vi "Get Variant Boxed Type Data Size.vi"(8 "error in (no error)":errorcluster, 11 "Data String":u8[](array[numeric])) -> (0 "error out":errorcluster, 2 "Data Size":i32, 3 "Remaining Data String":u8[](array[numeric]))   [LabVIEW 2017, in "Composition.lvlib"]
doc: "Determines the data size of the boxed type inside a variant.\n\n<B>Data Layout</B>\n[version][TD count][TDs][backref count][boxed data][number of attributes][attribute data][...]\n\nThe version part consists of four bytes, where the first part indicates the major LabVIEW version in Hexadecimal (e.g., [0x17, 0x00] = 2017) and the second part for the minor version of LabVIEW (e.g., [0x7f, 0x00] = SP1).\n\nTD count is four bytes indicating how many type definitions are packed in this variant part. What follows are the TDs, where the order of the TD in the set is important because TDs are re-used by index on the main type. For example, a cluster may have two strings. The string type only appears once and is referenced by the cluster twice. Note that types are always referenced, even if they are only used once.\n\nAfter the TDs, there are two bytes which (presumably) return the number of top-level types (so far, only 0x0001 was observed). After this comes the number of backref TDs (e.g., 0x0001 for the previous example of two strings in one cluster).\n\nThe backref TDs must be resolved in the primary TD to receive the \"original\" TD back. Effectively, uncompressing the variant. Here it is important to replace TDs at the right places in the primary TD (always from last to first to avoid replacing actual data).\n\nThe output of this is the unpacked type(s), which are passed as if they have been passed unpacked.\n\nNote that the same logic is used for attributes itself - recursively because an attribute can be a variant with attributes and so forth."
uses:
  Composition.lvlib
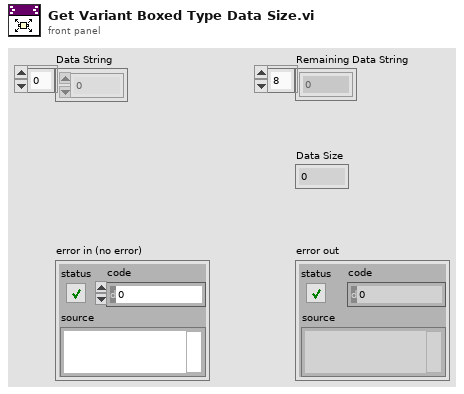
[diagram p1: front panel]
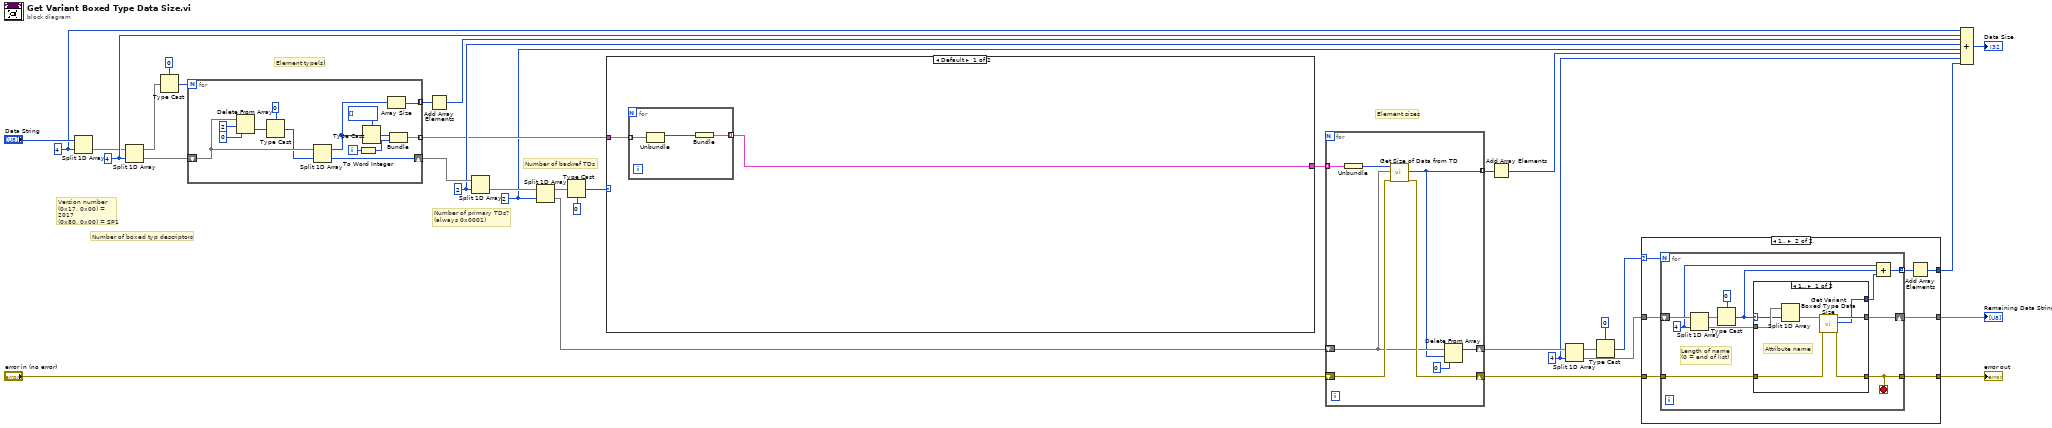
[diagram p0: block diagram]
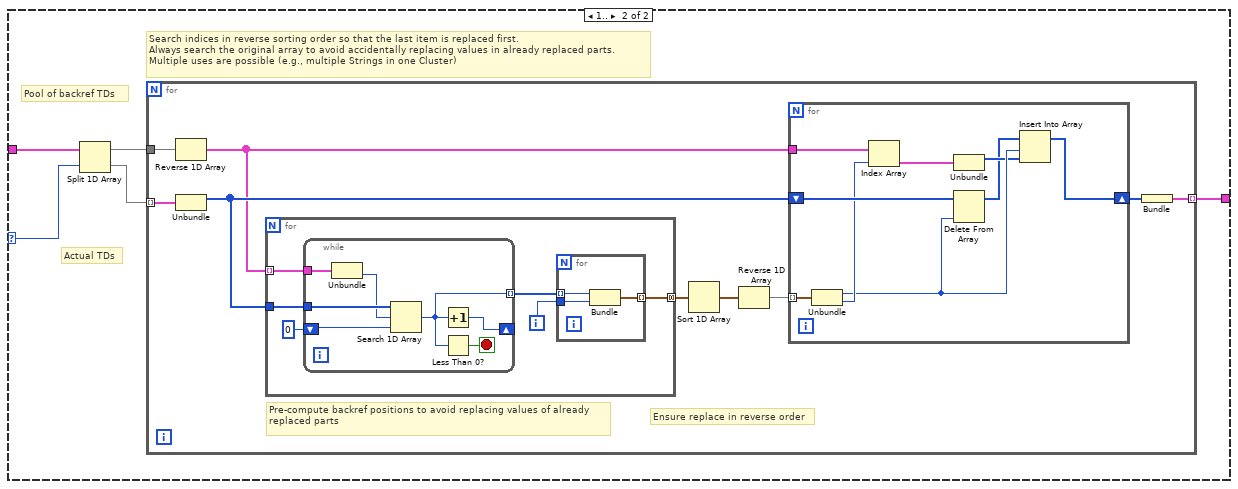
[diagram p4: hidden frame]
diagram:
  w8 = 4 ("index")
  w12 = 2 ("index")
  w26 = 2 ("length")
  w27 = 4 ("length")
  w28 = 4 ("length")
  # "Element sizes"
  # "Number of primary TDs?\n(always 0x0001)"
  # "Number of backref TDs"
  # "Version number\n(0x17, 0x00) = 2017\n(0x80, 0x00) = SP1"
  # "Element type(s)"
  # "Number of boxed typ descriptors"
  n1 = Split 1D Array(array="Data String", index=w28) -> (second subarray=w18:u8[])  [unwired: 1 out]
  n2 = Split 1D Array(array=w18, index=w27) -> (first subarray=w20:u8[], second subarray=w19:u8[])
  n3 = Type Cast(type=0 ("index"), x=w20) -> (*(type *) &x=w31:i32)
  n4 = for {
    N: w31 -> [_]
    shift-right: [w36] -> w30
    shift-left: w19 -> [w45]
    tunnel: [w42] -> w22 mode=indexing
    tunnel: [w39] -> w25 mode=indexing
    i -> [w38]
    n5 = Delete From Array(array=w45, length=2, index=0) -> (deleted portion=w47:u8[])  [unwired: 1 out]
    n6 = Type Cast(type=i16 0 ("index"), x=w47) -> (*(type *) &x=w44:i16)
    n7 = Split 1D Array(array=w45, index=w44) -> (first subarray=w35:u8[], second subarray=w36:u8[])
    n8 = To Word Integer(number=w38) -> (16bit integer=w37:i16)
    n9 = Type Cast(type=i16[] [] ("index"), x=w35) -> (*(type *) &x=w41:i16[])
    n10 = Array Size(array=w35) -> (size(s)=w39:i32)
    n11 = Bundle("index"=w41, w37) -> (w42:cluster{"index":i16[], i16})  [unwired: 1 in]
  }
  n12 = Add Array Elements(numeric array=w25) -> (sum=w24:i32)
  n13 = Split 1D Array(array=w30, index=w26) -> (second subarray=w15:u8[])  [unwired: 1 out]
  n14 = Split 1D Array(array=w15, index=w12) -> (first subarray=w13:u8[], second subarray=w14:u8[])
  n15 = Type Cast(type=i16 0 ("index"), x=w13) -> (*(type *) &x=w21:i16)
  n16 = case shown="Default" w21 {
    selector: w21 -> [_ w54]
    tunnel: w22 -> [w50 w58]
    tunnel: [w49 w55] -> w11
    frame Default {
      n17 = for {
        tunnel: w50 -> [w53] mode=indexing
        tunnel: [w51] -> w49 mode=indexing
        n18 = Unbundle(w53) -> ("index"=w52:i16[])  [unwired: 1 out]
        n19 = Bundle("index"=w52) -> (w51:cluster{"index":i16[]})  [unwired: 1 in]
      }
    }
    frame 1.. {
      # "Search indices in reverse sorting order so that the last item is replaced first.\nAlways search the original array to avoid accidentally replacing values in already replaced parts.\nMultiple uses are possible (e.g., multiple Strings in one Cluster)"
      # "Actual TDs"
      # "Pool of backref TDs"
      n20 = Split 1D Array(array=w58, index=w54) -> (first subarray=w56:cluster{"index":i16[], i16}[], second subarray=w57:cluster{"index":i16[], i16}[])
      n21 = for {
        tunnel: w57 -> [w66] mode=indexing
        tunnel: w56 -> [w67]
        tunnel: [w65] -> w55 mode=indexing
        # "Ensure replace in reverse order"
        # "Pre-compute backref positions to avoid replacing values of already replaced parts"
        n22 = Reverse 1D Array(array=w67) -> (reversed array=w62:cluster{"index":i16[], i16}[])
        n23 = Unbundle(w66) -> ("index"=w63:i16[])  [unwired: 1 out]
        n24 = for {
          tunnel: w62 -> [w72] mode=indexing
          tunnel: w63 -> [w73]
          tunnel: [w69] -> w61 mode=concatenating
          i -> [w70]
          n25 = while {
            tunnel: w73 -> [w83]
            tunnel: w72 -> [w82]
            tunnel: [w78] -> w71 mode=indexing
            shift-right: [w77] -> _
            shift-left: 0 -> [w79]
            stop <- w80 stop-if-true
            n26 = Unbundle(w82) -> (w81:i16)  [unwired: 1 out]
            n27 = Search 1D Array(1D array=w83, element=w81, start index (0)=w79) -> (index of element=w78:i32)
            n28 = Increment(x=w78) -> (x+1=w77:i32)
            n29 = Less Than 0?(x=w78) -> (x < 0?=w80:bool)
          }
          n30 = for {
            tunnel: w71 -> [w75] mode=indexing
            tunnel: w70 -> [w74]
            tunnel: [w76] -> w69 mode=indexing
            n31 = Bundle("index of element"=w75, w74) -> (w76:cluster{"index of element":i32, i32})  [unwired: 1 in]
          }
        }
        n32 = Sort 1D Array(array=w61) -> (sorted array=w60:cluster{"index of element":i32, i32}[])
        n33 = Reverse 1D Array(array=w60) -> (reversed array=w59:cluster{"index of element":i32, i32}[])
        n34 = for {
          tunnel: w62 -> [w89]
          shift-right: [w91] -> w64
          shift-left: w63 -> [w92]
          tunnel: w59 -> [w90] mode=indexing
          n35 = Unbundle(w90) -> ("index of element"=w86:i32, w87:i32)
          n36 = Index Array(array=w89, index=w87) -> (element=w88:cluster{"index":i16[], i16})
          n37 = Unbundle(w88) -> ("index"=w85:i16[])  [unwired: 1 out]
          n38 = Delete From Array(array=w92, index=w86) -> (array with subset deleted=w84:i16[])  [unwired: 1 in, 1 out]
          n39 = Insert Into Array(array=w84, index=w86, new element=w85) -> (w91:i16[])
        }
        n40 = Bundle("index"=w64) -> (w65:cluster{"index":i16[]})  [unwired: 1 in]
      }
    }
  }
  n41 = for {
    tunnel: [w96] -> w7 mode=indexing
    shift-right: [w99] -> w4
    shift-left: "error in (no error)" -> [w100]
    tunnel: w11 -> [w98] mode=indexing
    shift-right: [w95] -> w17
    shift-left: w14 -> [w97]
    n42 = Unbundle(w98) -> ("index"=w94:i16[])
    n43 = call "Get Size of Data from TD.vi"("error in (no error)"=w100, "Data String"=w97, "Type Descriptor"=w94) -> ("error out"=w99:errorcluster, "Size of Data"=w96:i32)  [unwired: 7 in]
    n44 = Delete From Array(array=w97, length=w96, index=0) -> (array with subset deleted=w95:u8[])  [unwired: 1 out]
  }
  n45 = Add Array Elements(numeric array=w7) -> (sum=w29:i32)
  n46 = Split 1D Array(array=w17, index=w8) -> (first subarray=w9:u8[], second subarray=w5:u8[])
  n47 = Type Cast(type=0 ("index"), x=w9) -> (*(type *) &x=w6:i32)
  n48 = case shown="1.." w6 {
    selector: w6 -> [_ w108]
    tunnel: w5 -> [w101 w109]
    tunnel: w4 -> [w102 w106]
    tunnel: [w102 w105] -> w3
    tunnel: [_ w104] -> w2
    tunnel: [w101 w103] -> w1
    frame Default {
    }
    frame 1.. {
      n49 = for {
        N: w108 -> [_]
        shift-right: [w120] -> w103
        shift-left: w109 -> [w119]
        tunnel: [w113] -> w107 mode=indexing
        tunnel: w106 -> [w115]
        tunnel: [w114] -> w105
        stop <- w114 stop-if-true
        w112 = 4 ("index")
        # "Length of name\n(0 = end of list)"
        n50 = Split 1D Array(array=w119, index=w112) -> (first subarray=w116:u8[], second subarray=w118:u8[])
        n51 = Type Cast(type=0 ("index"), x=w116) -> (*(type *) &x=w110:i32)
        n52 = case shown="1.." w110 {
          selector: w110 -> [w124 _]
          tunnel: [w123 w129] -> w120
          tunnel: w118 -> [w127 w129]
          tunnel: [w122 _] -> w111
          tunnel: w115 -> [w126 w128]
          tunnel: [w125 w128] -> w114
          frame 1.. {
            # "Attribute name"
            n53 = Split 1D Array(array=w127, index=w124) -> (second subarray=w121:u8[])  [unwired: 1 out]
            n54 = call "Get Variant Boxed Type Data Size.vi"("error in (no error)"=w126, "Data String"=w121) -> ("error out"=w125:errorcluster, "Data Size"=w122:i32, "Remaining Data String"=w123:u8[])  [unwired: 7 in]
          }
          frame Default {
          }
        }
        n55 = Compound Arithmetic op=ADD(w112, w110, w111) -> (w113:i32)
      }
      n56 = Add Array Elements(numeric array=w107) -> (sum=w104:i32)
    }
  }
  "error out" <- w3
  "Remaining Data String" <- w1
  n57 = Compound Arithmetic op=ADD(w28, w27, w24, w26, w12, w29, w8, w2) -> (→"Data Size":i32)
